vi "数值字符串转十六进制字符.vi"(11 "字符串输入":string) -> (3 "字符串输出":string)   [LabVIEW 2016, in "数据传输系统-06.lvlib"]
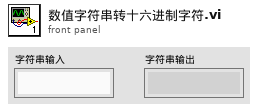
[diagram p1: front panel]
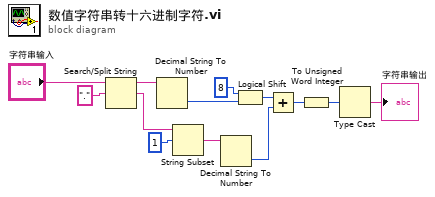
[diagram p0: block diagram]
diagram:
  n1 = Search/Split String(string="字符串输入", search string/char (-)="." ("搜索字符串/字符(-)")) -> (substring before match=w12:string, match + rest of string=w10:string)  [unwired: 1 in, 1 out]
  n2 = Decimal String To Number(string=w12) -> (number=w7:i32)  [unwired: 2 in, 1 out]
  n3 = String Subset(string=w10, offset (0)=1 ("偏移量(0)")) -> (substring=w13:string)  [unwired: 1 in]
  n4 = Decimal String To Number(string=w13) -> (number=w4:i32)  [unwired: 2 in, 1 out]
  n5 = Logical Shift(y=i16 8, x=w7) -> (x << y=w5:i32)
  n6 = Add(x=w5, y=w4) -> (x+y=w3:i32)
  n7 = To Unsigned Word Integer(number=w3) -> (unsigned 16bit integer=w2:u16)
  n8 = Type Cast(x=w2) -> (*(type *) &x=→"字符串输出":string)  [unwired: 1 in]
